vi "labview proje ödevi2.vi"() -> ()   [LabVIEW 2017]
uses:
  <vilib>/userdefined/High Color/IMAQdx.ctl
  <vilib>/vision/driver/NI_Vision_Acquisition_Software.lvlib
  <vilib>/vision/NI_Vision_Development_Module.lvlib
panel:
  out "error out 2":errorcluster
  out "Data":string
  out "Image":T1(plugin-control)
  out "Found?":bool
  out "error out":errorcluster
  in  "stop":bool
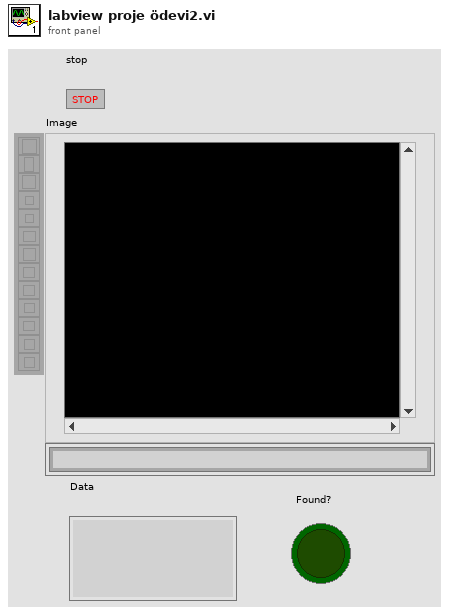
[diagram p1: front panel]
types:
  T1 = typedef "IMAQ Image.ctl" = refnum<image>
  T2 = typedef "IMAQdx.ctl" = refnum<k21>
  T3 = typedef "Image Type" = u32
  T4 = typedef "QR Code Report.ctl" = cluster{"Found?":bool, "Data":string, "Bounding Box":cluster{"x":sgl, "y":sgl}[], "Errors Corrected":u32, "Dimensions (Rows/Cols)":u32, "Version":u32, "QR Model":T5, "Stream Mode":T6, "Barcode Polarity":T7, "Mirrored?":bool, "Append Stream Position":u32, "Size of Append Stream":u32, "First EAN-128 ID":i32, "First Alternate Language ID":i32, "Append Stream ID":u32, "Minimum Edge Strength":u32, "Demodulation Mode":T8, "Cell Sample Size":T9, "Cell Filter Mode":T10}
  T5 = typedef "QR Code Model Type.ctl" = i32
  T6 = typedef "QR Code Stream Mode Type.ctl" = i32
  T7 = typedef "Data Matrix Polarity.ctl" = i32
  T8 = typedef "Demodulation Mode.ctl" = i32
  T9 = typedef "Cell Sample Size.ctl" = i32
  T10 = typedef "Cell Filter Mode.ctl" = i32
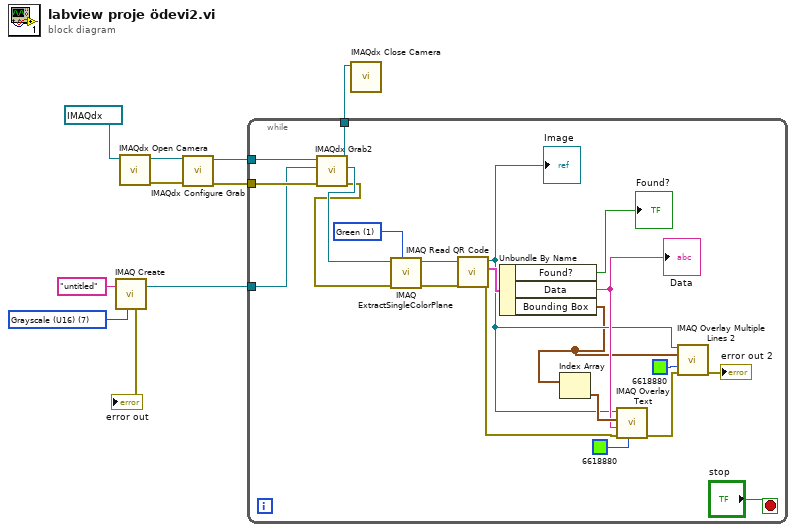
[diagram p0: block diagram]
diagram:
  w5 = T3 7 items=["Grayscale (U8)", "Grayscale (I16)", "Grayscale (SGL)", "Complex (CSG)", "RGB (U32)", "HSL (U32)", "RGB (U64)", "Grayscale (U16)"] ("Image Type")
  n1 = call "IMAQ Create"("Image Name"="untitled", "Image Type"=w5) -> ("New Image"=w3:T1, "error out"=→"error out":errorcluster)  [unwired: 3 in]
  n2 = call <vilib>:"IMAQdx Open Camera.vi"("Session In"=T2 "cam1") -> ("error out"=w9:errorcluster, "Session Out"=w10:T2)  [unwired: 9 in]
  n3 = call <vilib>:"IMAQdx Configure Grab.vi"("error in"=w9, "Session In"=w10) -> ("error out"=w7:errorcluster, "Session Out"=w8:T2)  [unwired: 8 in]
  n4 = while {
    tunnel: w8 -> [w30]
    tunnel: w7 -> [w29]
    tunnel: w3 -> [w12]
    tunnel: [w11] -> w2
    stop <- "stop" stop-if-true
    w28 = 1 items=["Red", "Green", "Blue", "Hue", "Saturation", "Luminance", "Value", "Intensity"] ("Color Plane")
    n5 = call <vilib>:"IMAQdx Grab2.vi"("error in"=w29, "Image In"=w12, "Session In"=w30) -> ("error out"=w24:errorcluster, "Image Out"=w25:T1, "Session Out"=w11:T2)  [unwired: 5 in, 1 out]
    n6 = call "IMAQ ExtractSingleColorPlane"("Color Plane"=w28, "error in (no error)"=w24, "Image Src"=w25) -> ("error out"=w26:errorcluster, "Image Dst Out"=w27:T1)  [unwired: 7 in]
    n7 = call "IMAQ Read QR Code"("error in (no error)"=w26, "Image"=w27) -> ("error out"=w13:errorcluster, "QR Code Report"=w23:T4, "Image (duplicate)"=w18:T1)  [unwired: 6 in, 1 out]
    "Image" <- w18
    n8 = Unbundle By Name(w23) -> ("Found?"=→"Found?":bool, "Data"=w20:string, "Bounding Box"=w17:cluster{"x":sgl, "y":sgl}[])
    "Data" <- w20
    n9 = Index Array(array=w17) -> (element=w21:cluster{"x":sgl, "y":sgl})  [unwired: 1 in]
    n10 = call "IMAQ Overlay Text"("Text Color (black)"=u32 6618880, "error in (no error)"=w13, "String"=w20, "Origin"=w21, "Image"=w18) -> ("error out"=w15:errorcluster)  [unwired: 5 in, 1 out]
    n11 = call "IMAQ Overlay Multiple Lines 2"("Image"=w18, "Line End Points"=w17, "Color"=u32 6618880, "error in (no error)"=w15) -> ("error out"=→"error out 2":errorcluster)  [unwired: 10 in, 1 out]
  }
  n12 = call <vilib>:"IMAQdx Close Camera.vi"("Session In"=w2) -> ()  [unwired: 10 in, 1 out]
